vi "Actor Core.vi"(8 "error in":errorcluster, 11 "Range Controller Actor in":refnum<class "Range Controller Actor.lvclass">) -> (0 "error out":errorcluster, 3 "Actor out":refnum<class "Actor.lvclass">)   [LabVIEW 2018, in "Range Controller.lvlib" / "Range Controller Actor.lvclass"]
doc: "(<B>Filename</B>: Actor Framework.lvlib:Actor.lvclass:Actor Core.vi)\n\nReceives messages to the actor, reacts to them, and initiates any error handling that may shut the actor down.\n\nDescendant classes may override this VI to append parallel tasks for the actor to complete while it handles messages. Overrides use the Call Parent Method node."
uses:
  Range Controller Actor.lvclass
  C:/Program Files (x86)/National Instruments/LabVIEW 2018/vi.lib/ActorFramework/Actor/Actor.lvclass
  <vilib>/ActorFramework/Actor/Actor.lvclass
  <vilib>/ActorFramework/Actor/Actor.lvclass/Actor.ctl
  <vilib>/ActorFramework/Message Enqueuer/Message Enqueuer.lvclass/Message Enqueuer.ctl
  Range Controller Actor.lvclass/Range Controller Actor.ctl
  <vilib>/ActorFramework/Message Enqueuer/Init from Existing Queue.vi
  <vilib>/ActorFramework/Message Enqueuer/Enqueue.vi
  <vilib>/ActorFramework/Stop Msg/Stop Msg.lvclass
  C:/Program Files (x86)/National Instruments/LabVIEW 2018/vi.lib/ActorFramework/Message/Message.lvclass
  <vilib>/ActorFramework/Message Priority Queue/Priority Enqueue.vi
  Actor Monitor/Actor/Monitored Actor.lvclass
  <vilib>/ActorFramework/Message Enqueuer/Message Enqueuer.lvclass
  Range Controller Actor Messages/Check Deadband Msg/Check Deadband Msg.lvclass
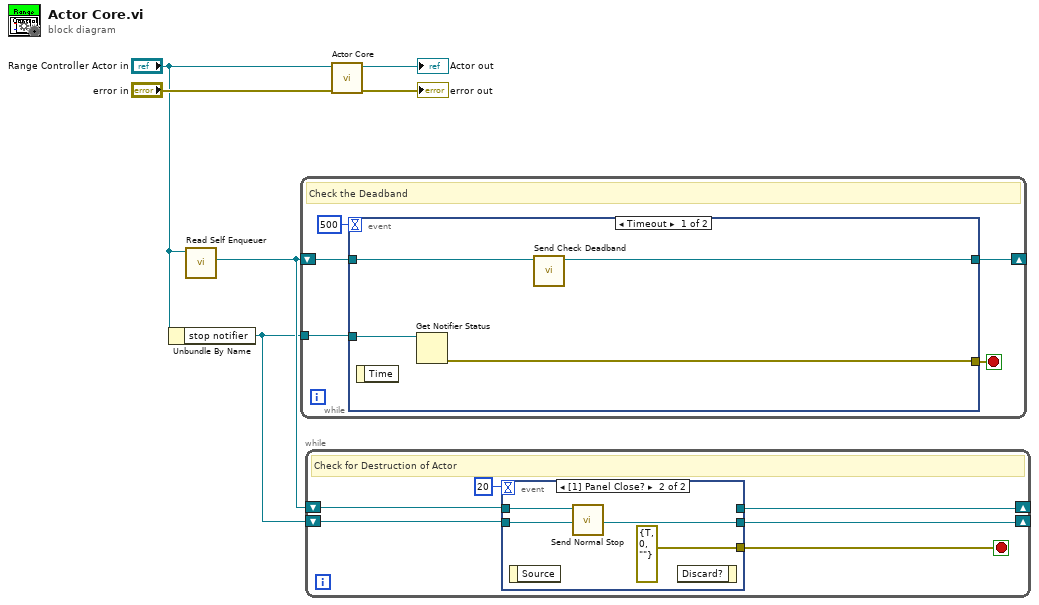
[diagram p0: block diagram]
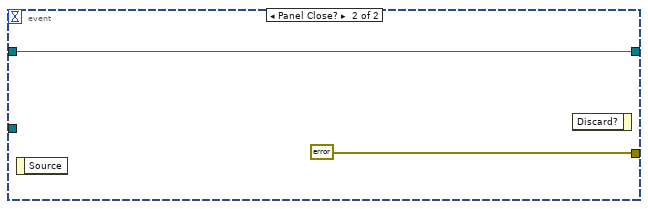
[diagram p2: hidden frame]
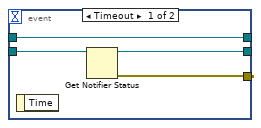
[diagram p3: hidden frame]
diagram:
  n1 = Unbundle By Name("Range Controller Actor in") -> ("stop notifier"=w1:refnum<notifier>)
  n2 = call <vilib>:"Read Self Enqueuer.vi"("Actor"="Range Controller Actor in") -> ("Self Enqueuer"=w2:refnum<class "Message Enqueuer.lvclass">)  [unwired: 10 in]
  n3 = while {
    tunnel: w1 -> [w11]
    shift-right: [w7] -> _
    shift-left: w2 -> [w8]
    stop <- w9 stop-if-true
    # "Check the Deadband"
    n4 = event shown="[0] Timeout" {
      selector: _ -> [_ _]
      dyn-events: _ -> [_ _]
      timeout: 500 -> [_ _]
      tunnel: w11 -> [w15 _]
      tunnel: [w14 errorcluster {"status"=TRUE, "code"=0, "source"=""} ("error out")] -> w9
      tunnel: w8 -> [w13 w16]
      tunnel: [w12 w16] -> w7
      event Timeout {
        n5 = event-data() -> ()  [unwired: 1 in, 1 out]
        n6 = Get Notifier Status(notifier=w15) -> (error out=w14:errorcluster)  [unwired: 1 in, 4 out]
        n7 = call "Send Check Deadband.vi"("Message Enqueuer in"=w13) -> ("Message Enqueuer out"=w12:refnum<class "Message Enqueuer.lvclass">)  [unwired: 9 in, 1 out]
      }
      event Panel Close? {
        n8 = event-data() -> ()  [unwired: 1 in, 1 out]
        n9 = event-data() -> ()  [unwired: 2 in, 1 out]
      }
    }
  }
  n10 = while {
    shift-right: [w19] -> _
    shift-left: w2 -> [w20]
    shift-right: [w18] -> _
    shift-left: w1 -> [w23]
    stop <- w21 stop-if-true
    # "Check for Destruction of Actor"
    n11 = event shown="[1] Panel Close?" {
      selector: _ -> [_ _]
      dyn-events: _ -> [_ _]
      timeout: 20 -> [_ _]
      tunnel: w23 -> [w27 w29]
      tunnel: [w26 errorcluster {"status"=TRUE, "code"=0, "source"=""} ("error out")] -> w21
      tunnel: w20 -> [w25 w28]
      tunnel: [w25 _] -> w19
      tunnel: [w24 w29] -> w18
      event Timeout {
        n12 = event-data() -> ()  [unwired: 1 in, 1 out]
        n13 = Get Notifier Status(notifier=w27) -> (notifier out=w24:refnum<notifier>, error out=w26:errorcluster)  [unwired: 1 in, 3 out]
      }
      event Panel Close? {
        n14 = event-data() -> ()  [unwired: 1 in, 1 out]
        n15 = call <vilib>:"Send Normal Stop.vi"("Message Enqueuer"=w28) -> ()  [unwired: 10 in, 1 out]
        n16 = event-data() -> ()  [unwired: 2 in, 1 out]
      }
    }
  }
  n17 = call-parent "Actor Core.vi"("error in"="error in", "Actor in"="Range Controller Actor in") -> ("error out"=→"error out":errorcluster, "Actor out"=→"Actor out":refnum<class "Actor.lvclass">)  [unwired: 8 in]
